vi "Build_Asylum_SetInWavePair.vi"(4 "decimation":i32, 6 "callback":string, 7 "whichBank":i32, 8 "error in (no error)":errorcluster, 9 "WaveB":cluster{"channelStringB":string, "waveB":string}, 10 "WaveA":cluster{"channelStringA":string, "waveA":string}, 11 "eventString":string) -> (0 "error out":errorcluster, 3 "Command":string)   [LabVIEW 2019]
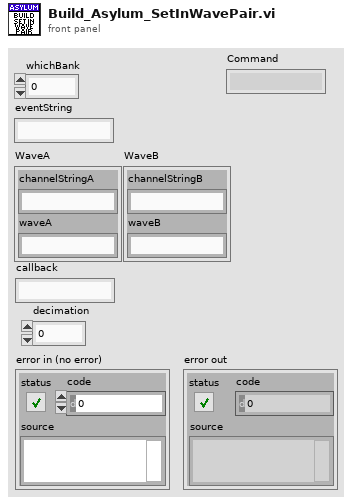
[diagram p1: front panel]
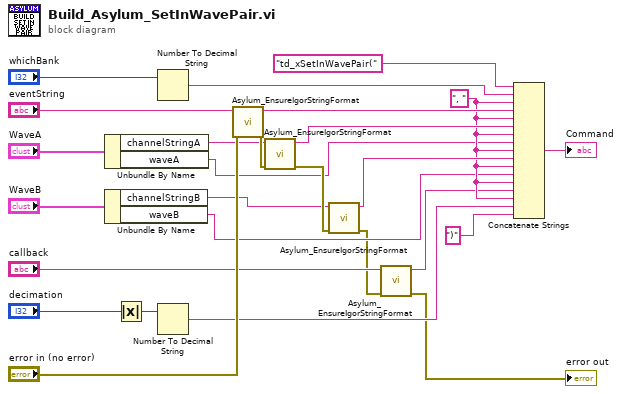
[diagram p0: block diagram]
diagram:
  w10 = ", "
  n1 = Unbundle By Name("WaveA") -> ("channelStringA"=w23:string, "waveA"=w5:string)
  n2 = Unbundle By Name("WaveB") -> ("channelStringB"=w14:string, "waveB"=w6:string)
  n3 = Absolute Value(x="decimation") -> (abs(x)=w22:i32)
  n4 = Number To Decimal String(number="whichBank") -> (decimal integer string=w20:string)  [unwired: 1 in]
  n5 = Number To Decimal String(number=w22) -> (decimal integer string=w9:string)  [unwired: 1 in]
  n6 = call "Asylum_EnsureIgorStringFormat.vi"("error in (no error)"="error in (no error)", "Value"="eventString") -> ("error out"=w26:errorcluster, "Value"=w19:string)  [unwired: 8 in]
  n7 = call "Asylum_EnsureIgorStringFormat.vi"("error in (no error)"=w26, "Value"=w23) -> ("error out"=w24:errorcluster, "Value"=w18:string)  [unwired: 8 in]
  n8 = call "Asylum_EnsureIgorStringFormat.vi"("error in (no error)"=w24, "Value"=w14) -> ("error out"=w2:errorcluster, "Value"=w11:string)  [unwired: 8 in]
  n9 = call "Asylum_EnsureIgorStringFormat.vi"("error in (no error)"=w2, "Value"="callback") -> ("error out"=→"error out":errorcluster, "Value"=w3:string)  [unwired: 8 in]
  n10 = Concatenate Strings("td_xSetInWavePair(" ("string"), w20, w10, w19, w10, w18, w10, w5, w10, w11, w10, w6, w10, w3, w10, w9, ")" ("string")) -> (→"Command":string)
